vi "DAQmx Create Channel (AI-Sound Pressure-Microphone).vi"(0 "task in":refnum<k21>, 1 "maximum sound pressure level":dbl=100.0 format="%0.2f", 3 "input terminal configuration":i32(ring)=-1 items=["default"=-1, "RSE"=10083, "NRSE"=10078, "Differential"=10106, "Pseudodifferential"=12529], 5 "physical channels":tag, 6 "current excitation source":i32(ring)=10200 items=["Internal"=10200, "External"=10167, "None"=10230], 7 "name to assign":string, 8 "current excitation value":dbl=0.004, 9 "units":i32(ring)=10081 items=["Pascals"=10081, "From Custom Scale"=10065], 11 "error in":errorcluster, 12 "custom scale name":tag, 13 "microphone sensitivity":dbl=10.0) -> (4 "task out":refnum<k21>, 15 "error out":errorcluster)   [LabVIEW 2011]
doc: "Creates channel(s) that use a microphone to measure sound pressure."
uses:
  C:/Program Files/National Instruments/LabVIEW 2011/resource/objmgr/daqmx.rc
panel:
  # "input limits"
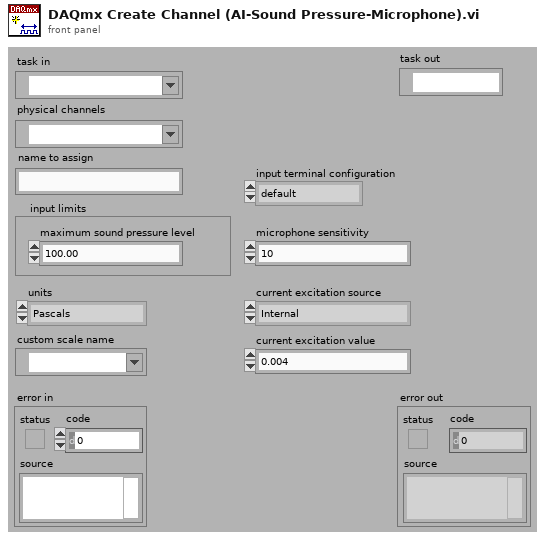
[diagram p1: front panel]
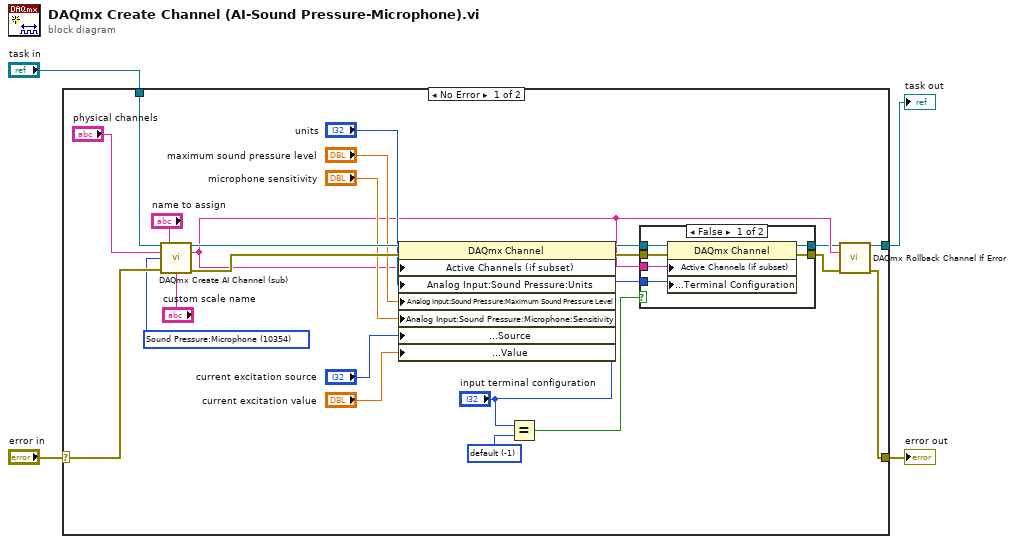
[diagram p0: block diagram]
diagram:
  n1 = case shown="No Error" "error in" {
    selector: "error in" -> [w25 w37]
    tunnel: [w19 w37] -> w2
    tunnel: "task in" -> [w26 w36]
    tunnel: [w20 w36] -> w1
    frame No Error {
      w9 = -1 items=["default"=-1, "differential"=10106, "RSE"=10083, "NRSE"=10078] ("input terminal configuration")
      w15 = 10354 items=["Voltage"=10322, "Current"=10134, "More:Voltage:Custom with Excitation"=10323, "More:Current:Custom with Excitation"=10136, "Frequency"=10181, "Period"=10257, "Resistance"=10278, "Temperature:Thermocouple"=10303, "Temperature:Thermistor"=10302, "Temperature:RTD"=10301, "Temperature:Built-in Sensor"=10311, "Strain Gage"=10300, "LVDT"=10352, "RVDT"=10353, "Accelerometer:Voltage Input"=10355, "Accelerometer:Current Input"=10356, "Sound Pressure:Microphone"=10354] ("measurement type")
      n2 = call "DAQmx Create AI Channel (sub).vi"("task in"=w26, "virtual channel name"="name to assign", "physical channel name"="physical channels", "measurement type"=w15, "error in"=w25, "custom scale"="custom scale name") -> ("task out"=w27:refnum<k21>, "channel names"=w10:string, "error out"=w22:errorcluster)  [unwired: 1 in, 6 out]
      n3 = property class="DAQmx Channel"(reference=w27, error in=w22, "Active Channels (if subset)"=w10, "Analog Input:Sound Pressure:Units"="units", "Analog Input:Sound Pressure:Maximum Sound Pressure Level"="maximum sound pressure level", "Analog Input:Sound Pressure:Microphone:Sensitivity"="microphone sensitivity", "Analog Input:General Properties:Signal Conditioning:Excitation:Source"="current excitation source", "Analog Input:General Properties:Signal Conditioning:Excitation:Value"="current excitation value") -> (reference out=w12:refnum<k21>, error out=w11:errorcluster)
      n4 = Equal?(x="input terminal configuration", y=w9) -> (x = y?=w8:bool)
      n5 = case shown="False" w8 {
        tunnel: w11 -> [w33 w35]
        tunnel: [w32 w34] -> w6
        tunnel: [w31 w35] -> w5
        tunnel: "input terminal configuration" -> [w30 _]
        tunnel: w10 -> [w29 _]
        tunnel: w12 -> [w28 w34]
        frame False {
          n6 = property class="DAQmx Channel"(reference=w28, error in=w33, "Active Channels (if subset)"=w29, "Analog Input:General Properties:Input Configuration:Terminal Configuration"=w30) -> (reference out=w32:refnum<k21>, error out=w31:errorcluster)
        }
        frame True {
        }
      }
      n7 = call "DAQmx Rollback Channel If Error.vi"("task in"=w6, "channel names"=w10, "error in"=w5) -> ("task out"=w20:refnum<k21>, "error out"=w19:errorcluster)  [unwired: 11 out]
    }
    frame Error {
    }
  }
  "error out" <- w2
  "task out" <- w1
